vi "ExEasyEm.vi"(5 "Easy EM  Mode":bool, 6 "Em Gain":dbl format="%.2f", 7 "error in (no error)":errorcluster) -> (0 "Em Gain Value for 10 Mhz":dbl format="%.2f", 1 "Em Gain Value for 20 Mhz":dbl format="%.2f", 2 "Em Gain Value for 40 Mhz":dbl format="%.2f", 3 "error out":errorcluster, 4 "Em Gain":dbl format="%.2f")   [LabVIEW 2010]
uses:
  Open-Close/CamHandle.vi
panel:
  # "ExEasyEm.vi : this Vi shows how to control the Easy EM mode and the EM Gain used in \nQ-Imaging cameras. If the Easy EM Mode is set then the EM Gain is inactive"
  # "NOTICE\n\nTHIS VI USES A GLOBAL CAMERA HANDLE\n\nTHE VI EXOPENGLOBALCAM.VI MUST BE\nRUN AT THE START OF THE WORK SESSION.\nTHE CAMERA WILL REMAIN OPENED.\n\nTHE VI EXCLOSEGLOBALCAM.VI MUST\nBE RUN BEFORE LEAVING LABVIEW."
  # "Note: this is inactive if Em Gain Mode or Em Gain Locked are set."
  # "Note: This example requires Q imaging\ndrivers 2.0.9 or greater"
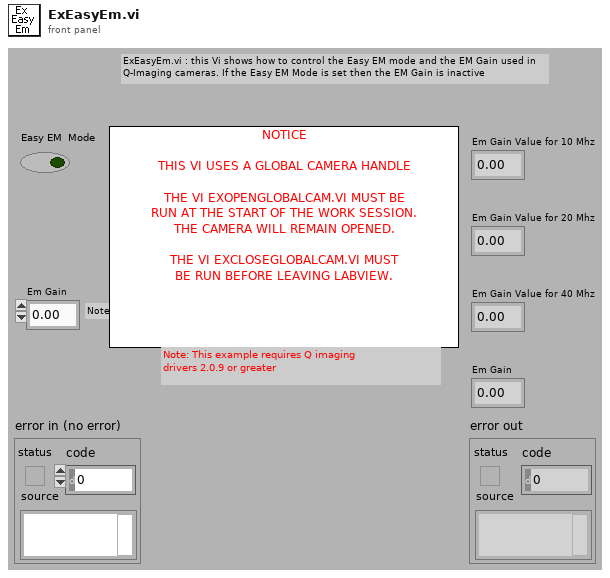
[diagram p1: front panel]
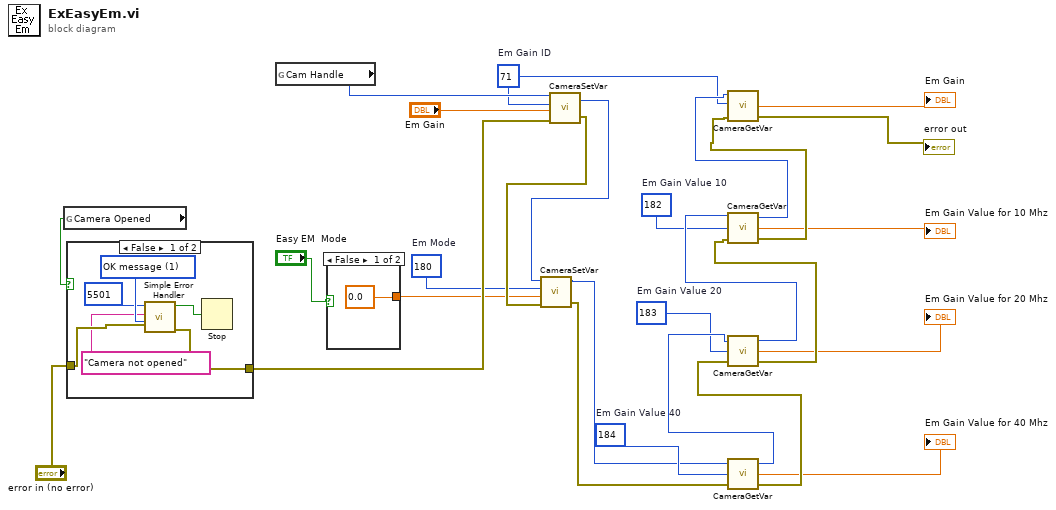
[diagram p0: block diagram]
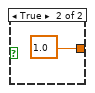
[diagram p2: hidden frame]
diagram:
  w3 = 184  # Em Gain Value 40
  w4 = 183  # Em Gain Value 20
  w5 = 182  # Em Gain Value 10
  w12 = 180  # Em Mode
  w14 = 71  # Em Gain ID
  n1 = global read "CamHandle.vi" "Camera Opened"() -> (w27:bool)
  n2 = case shown="False" w27 {
    tunnel: "error in (no error)" -> [w32 w34]
    tunnel: [w31 w34] -> w23
    frame False {
      w33 = u16 1 items=["no dialog", "OK message", "continue or stop message"] ("type of dialog (OK msg:1)")
      n3 = call <vilib>:"Simple Error Handler.vi"("error code (no error:0)"=5501, "error source (\" \")"="Camera not opened", "type of dialog (OK msg:1)"=w33, "error in (no error)"=w32) -> ("error?"=w29:bool, "error out"=w31:errorcluster)  [unwired: 1 in, 3 out]
      n4 = Stop(stop? (T)=w29) -> ()
    }
    frame True {
    }
  }
  n5 = global read "CamHandle.vi" "Cam Handle"() -> (w25:u32)
  n6 = case shown="False" "Easy EM  Mode" {
    tunnel: [0.0 1.0] -> w11
    frame False {
    }
    frame True {
    }
  }
  n7 = call <userlib>:"CameraSetVar.vi"("error in"=w23, "Value"="Em Gain", "Parameter ID"=w14, "Camera Handle"=w25) -> ("error out"=w22:errorcluster, "CameraHandle"=w24:u32)
  n8 = call <userlib>:"CameraSetVar.vi"("error in"=w22, "Value"=w11, "Parameter ID"=w12, "Camera Handle"=w24) -> ("error out"=w1:errorcluster, "CameraHandle"=w2:u32)
  n9 = call <userlib>:"CameraGetVar.vi"("error in"=w1, "Parameter ID"=w3, "Camera Handle"=w2) -> ("error out"=w20:errorcluster, "Value"=→"Em Gain Value for 40 Mhz":dbl, "Camera Handle"=w21:u32)
  n10 = call <userlib>:"CameraGetVar.vi"("error in"=w20, "Parameter ID"=w4, "Camera Handle"=w21) -> ("error out"=w18:errorcluster, "Value"=→"Em Gain Value for 20 Mhz":dbl, "Camera Handle"=w19:u32)
  n11 = call <userlib>:"CameraGetVar.vi"("error in"=w18, "Parameter ID"=w5, "Camera Handle"=w19) -> ("error out"=w16:errorcluster, "Value"=→"Em Gain Value for 10 Mhz":dbl, "Camera Handle"=w17:u32)
  n12 = call <userlib>:"CameraGetVar.vi"("error in"=w16, "Parameter ID"=w14, "Camera Handle"=w17) -> ("error out"=→"error out":errorcluster, "Value"=→"Em Gain":dbl)  [unwired: 1 out]
